vi "Add Event Reference to maps.vi"(7 "New Node Path":string, 8 "Event type":T1, 9 "Event VIs":refnum<vi>[](array[refnum]), 10 "Tree Map in":T2, 11 "map ref in":map{string, refnum<vi>}(c390)) -> (2 "Tree Map out":T2, 3 "map ref out":map{string, refnum<vi>}(c390))   [LabVIEW 2020, in "Panther Dashboard.lvlib"]
uses:
  Panther Dashboard.lvlib
  <vilib>/National Instruments/Tree Map/Tree Map Data.ctl
  Event types--enum.ctl
  <vilib>/National Instruments/Tree Map/Tree Map.lvlib
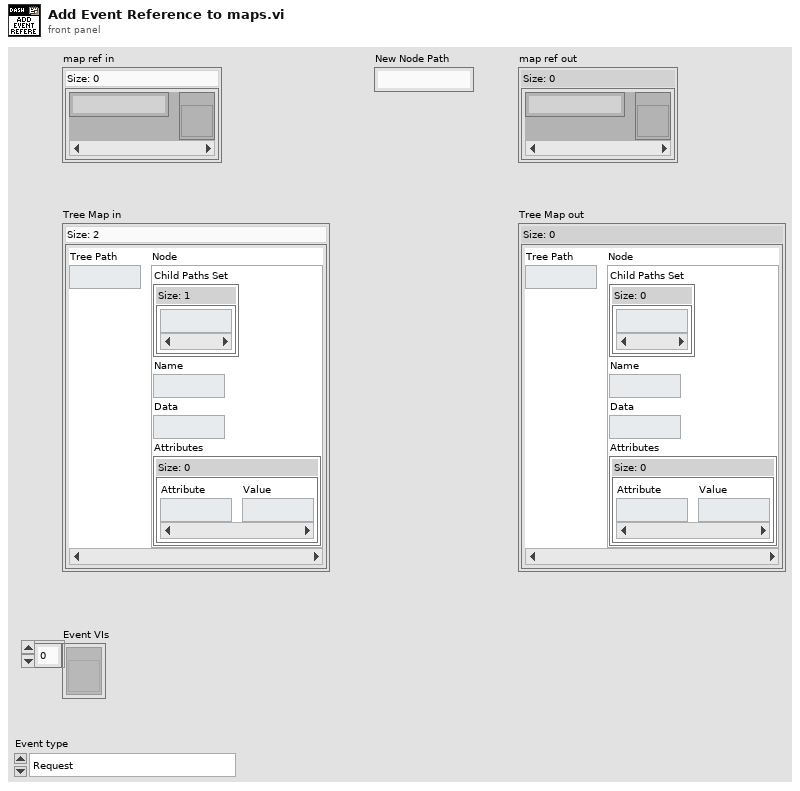
[diagram p1: front panel]
types:
  T1 = typedef "Panther Dashboard.lvlib/Event types--enum.ctl" = enum16{"Request", "Request and Wait for Reply", "Broadcast"}
  T2 = typedef "Tree Map.lvlib/Tree Map Data.ctl" = map{string, cluster{"Child Paths Set":set{string}, "Name":string, "Data":string, "Attributes":map{string, string}}}
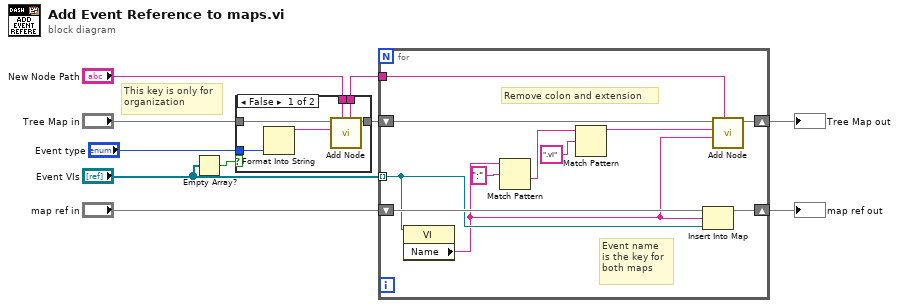
[diagram p0: block diagram]
diagram:
  # "This key is only for\norganization"
  n1 = Empty Array?(array="Event VIs") -> (empty?=w1:bool)
  n2 = case shown="False" w1 {
    tunnel: "New Node Path" -> [w15 w18]
    tunnel: [w14 w18] -> w6
    tunnel: "Tree Map in" -> [w13 w17]
    tunnel: [w12 w17] -> w4
    tunnel: "Event type" -> [w11 _]
    frame False {
      n3 = Format Into String(w11) -> (resulting string=w16:string)  [unwired: 3 in, 1 out]
      n4 = call <vilib>:"Add Node.vi"("Parent Path"=w15, "New Node Name"=w16, "Tree Map In"=w13) -> ("Tree Map Out"=w12:T2, "New Node Path"=w14:string)  [unwired: 6 in, 1 out]
    }
    frame True {
    }
  }
  n5 = for {
    tunnel: w6 -> [w29]
    shift-right: [w27] -> w10
    shift-left: w4 -> [w28]
    shift-right: [w25] -> w8
    shift-left: "map ref in" -> [w26]
    tunnel: "Event VIs" -> [w20] mode=indexing
    # "Event name\nis the key for \nboth maps"
    # "Remove colon and extension"
    n6 = property class="VI"(reference=w20) -> ("Name"=w19:string)  [unwired: 1 in, 2 out]
    n7 = Match Pattern(string=w19, regular expression=":") -> (after substring=w22:string)  [unwired: 1 in, 3 out]
    n8 = Match Pattern(string=w22, regular expression=".vi") -> (before substring=w21:string)  [unwired: 1 in, 3 out]
    n9 = Insert Into Map(map in=w26, key=w19, value=w20) -> (map out=w25:map{string, refnum<vi>})  [unwired: 2 out]
    n10 = call <vilib>:"Add Node.vi"("Parent Path"=w29, "Data"=w19, "New Node Name"=w21, "Tree Map In"=w28) -> ("Tree Map Out"=w27:T2)  [unwired: 5 in, 2 out]
  }
  "Tree Map out" <- w10
  "map ref out" <- w8
